vi "Command Channel.vi"(8 "error in":errorcluster, 11 "Node Ptr":T1 format="%.0x") -> (0 "error out":errorcluster)   [LabVIEW 2020, in "Ballard MIL-STD-1553 System Explorer.lvlib" / "Implementation.lvlib"]
uses:
  Implementation.lvlib
  <vilib>/NI VeriStand/Custom Device API/Custom Device Item Ref.ctl
  <vilib>/NI VeriStand/Custom Device API/Custom Device Channel Type.ctl
  <vilib>/NI VeriStand/Custom Device API/Custom Device API.lvlib
panel:
  out "Channel Settings":string[][](table)
  in  "Default Value":dbl
  in  "SHDocVw.IWebBrowser":refnum<k7>(container)
  in  "General Header":cluster{"Section Name":string}={"Section Name"="Ballard MIL-STD 1553 - Command Channel"}
  in  "Description":string
  out "Name":string
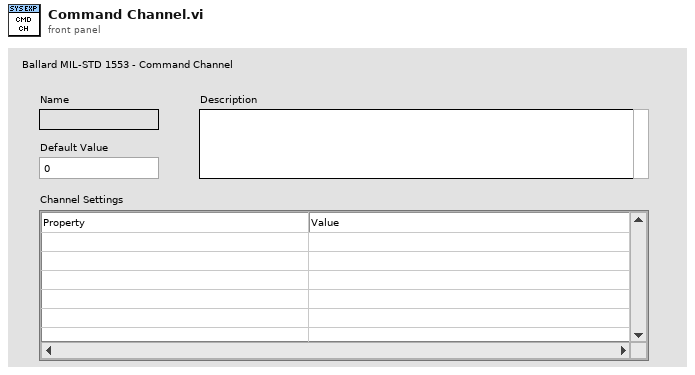
[diagram p1: front panel]
types:
  T1 = typedef "Custom Device API.lvlib/Custom Device Item Ref.ctl" = u64
  T2 = typedef "Custom Device API.lvlib/Custom Device Channel Type.ctl" = enum16{"Input", "Output"}
  T3 = typedef "Custom Device API.lvlib/Custom Device Channel.ctl" = cluster{"Type":T2, "Units":string, "Default Value":dbl, "Faultable":bool, "Scalable":bool}
  T4 = typedef "Custom Device API.lvlib/Custom Device Commands.ctl" = enum16{"Default", "Item renamed", "Shutdown", "Dynamic button pressed"}
  T5 = typedef "Custom Device API.lvlib/Custom Device Item Info.ctl" = cluster{"Name":string, "Is Channel":bool, "GUID":string, "Is Waveform":bool}
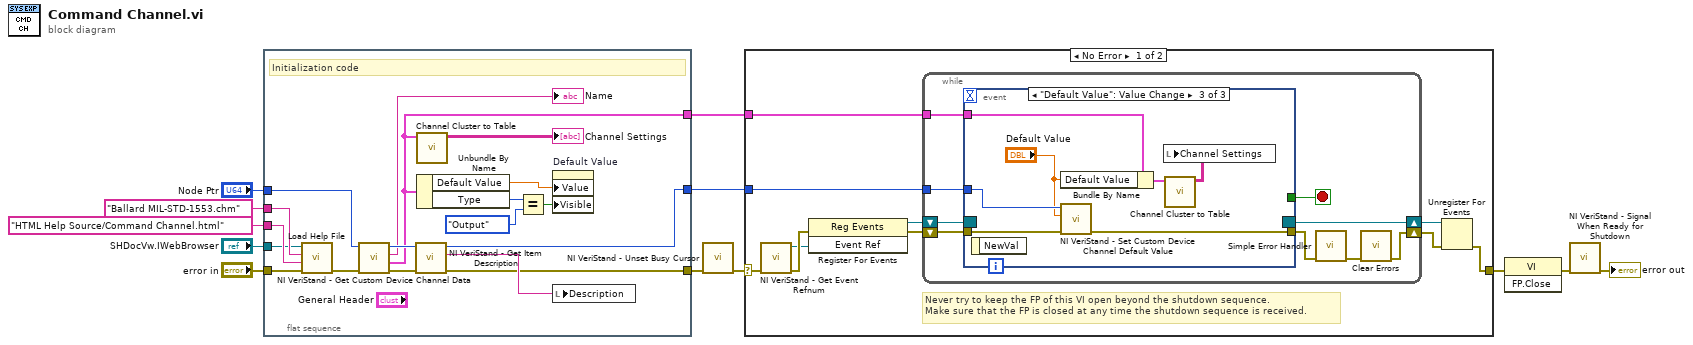
[diagram p0: block diagram]
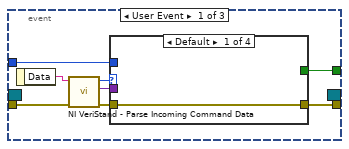
[diagram p2: hidden frame]
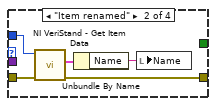
[diagram p3: hidden frame]
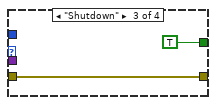
[diagram p4: hidden frame]
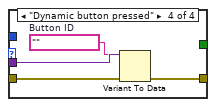
[diagram p5: hidden frame]
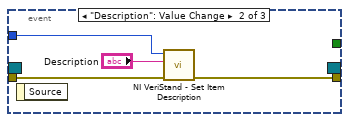
[diagram p6: hidden frame]
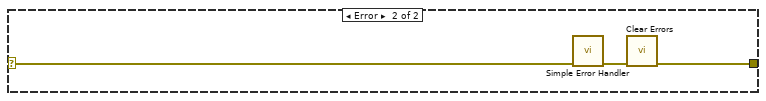
[diagram p7: hidden frame]
diagram:
  n1 = flat-sequence "Initialization code" {
    tunnel: "error in" -> [w29]
    tunnel: "Node Ptr" -> [w25]
    tunnel: [w24] -> w8
    tunnel: [w23] -> w5
    tunnel: "SHDocVw.IWebBrowser" -> [w26]
    tunnel: "HTML Help Source/Command Channel.html" ("CD_CHM_Section") -> [w28]
    tunnel: "Ballard MIL-STD-1553.chm" ("CD_CHM_FileName") -> [w27]
    tunnel: [w13] -> w1
    frame #0 {
      # "Initialization code"
      n2 = call "Load Help File.vi"("error in (no error)"=w29, "HTML File to Load"=w28, "Main CHM File"=w27, "Browser"=w26) -> ("error out"=w21:errorcluster)  [unwired: 7 in]
      n3 = call <vilib>:"NI VeriStand - Get Custom Device Channel Data.vi"("error in (no error)"=w21, "Channel Ref in"=w25) -> ("error out"=w22:errorcluster, "Channel"=w13:T3, "Channel Name"=→"Name":string, "Channel Ref out"=w17:T1)  [unwired: 4 in, 2 out]
      n4 = call <vilib>:"NI VeriStand - Get Item Description.vi"("error in (no error)"=w22, "Item Ref in"=w17) -> ("error out"=w24:errorcluster, "Description"=w30:string, "Item Ref out"=w23:T1)  [unwired: 7 out]
      n5 = call "Channel Cluster to Table.vi"("channel settings"=w13) -> ("channel settings table"=→"Channel Settings":string[][])  [unwired: 10 in]
      n6 = Unbundle By Name(w13) -> ("Default Value"=w14:dbl, "Type"=w20:T2)
      n7 = Equal?(x=w20, y=Custom_Device_Channel_Type."Output" ("x")) -> (x = y?=w18:bool)
      n8 = property on="Default Value" class="DigNum (strict)"("Value"=w14, "Visible"=w18) -> ()  [unwired: 2 in, 2 out]
      n9 = local write "Description"(w30) -> ()
    }
  }
  n10 = call <vilib>:"NI VeriStand - Unset Busy Cursor.vi"("error in (no error)"=w8) -> ("error out"=w7:errorcluster)  [unwired: 10 out]
  n11 = case shown="No Error" w7 {
    selector: w7 -> [w32 w83]
    tunnel: [w37 w81] -> w12
    tunnel: w5 -> [w33 _]
    tunnel: w1 -> [w31 _]
    frame No Error {
      # "Never try to keep the FP of this VI open beyond the shutdown sequence.\nMake sure that the FP is closed at any time the shutdown sequence is received."
      n12 = call <vilib>:"NI VeriStand - Get Event Refnum.vi"("error in (no error)"=w32) -> ("error out"=w40:errorcluster, "Event Ref"=w36:refnum<user-event>)  [unwired: 9 out]
      n13 = register-events(error in=w40, w36) -> (reference out=w34:refnum<event-registration>, error out=w35:errorcluster)  [unwired: 1 in]
      n14 = while {
        tunnel: w33 -> [w45]
        shift-right: [w42] -> w38
        shift-left: w35 -> [w48]
        shift-right: [w49] -> w39
        shift-left: w34 -> [w47]
        tunnel: w31 -> [w41]
        stop <- w46 stop-if-true
        n15 = event shown="[2] \"Default Value\": Value Change" {
          selector: w47 -> [_ _ _]
          dyn-events: [_ _ _] -> w49
          timeout: _ -> [_ _ _]
          tunnel: w48 -> [w57 w72 w80]
          tunnel: [w54 _ _] -> w46
          tunnel: [w53 w71 w79] -> w44
          tunnel: w45 -> [w52 w73 w78]
          tunnel: w41 -> [_ _ w76]
          event User Event {
            n16 = event-data() -> ("Data"=w50:string)  [unwired: 1 out]
            n17 = call <vilib>:"NI VeriStand - Parse Incoming Command Data.vi"("error in (no error)"=w57, "Incoming data"=w50) -> ("error out"=w56:errorcluster, "Outgoing data"=w51:variant, "Action"=w55:T4)  [unwired: 7 out]
            n18 = case shown="Default" w55 {
              tunnel: w56 -> [w58 w63 w64 w69]
              tunnel: [_ _ TRUE _] -> w54
              tunnel: [w58 w60 w64 w66] -> w53
              tunnel: w52 -> [_ w62 _ _]
              tunnel: w51 -> [_ _ _ w68]
              frame Default {
              }
              frame "Item renamed" {
                n19 = call <vilib>:"NI VeriStand - Get Item Data.vi"("error in (no error)"=w63, "Item Ref in"=w62) -> ("error out"=w60:errorcluster, "Item Info"=w61:T5)  [unwired: 8 out]
                n20 = Unbundle By Name(w61) -> ("Name"=w59:string)
                n21 = local write "Name"(w59) -> ()
              }
              frame "Shutdown" {
              }
              frame "Dynamic button pressed" {
                w67 = ""  # Button ID
                n22 = Variant To Data(error in=w69, type=w67, Variant=w68) -> (error out=w66:errorcluster)  [unwired: 1 out]
              }
            }
          }
          event "Description": Value Change {
            n23 = event-data() -> ()  [unwired: 2 out]
            n24 = call <vilib>:"NI VeriStand - Set Item Description.vi"("error in (no error)"=w72, "Description"="Description", "Item Ref in"=w73) -> ("error out"=w71:errorcluster)  [unwired: 8 out]
          }
          event "Default Value": Value Change {
            n25 = event-data() -> ()  [unwired: 2 out]
            n26 = Bundle By Name(cluster=w76, "Default Value"="Default Value") -> (w74:T3)
            n27 = call <vilib>:"NI VeriStand - Set Custom Device Channel Default Value.vi"("error in (no error)"=w80, "Default Value"="Default Value", "Channel Ref in"=w78) -> ("error out"=w79:errorcluster)  [unwired: 7 in, 1 out]
            n28 = call "Channel Cluster to Table.vi"("channel settings"=w74) -> ("channel settings table"=w77:string[][])  [unwired: 10 in]
            n29 = local write "Channel Settings"(w77) -> ()
          }
        }
        n30 = call <vilib>:"Simple Error Handler.vi"("error in (no error)"=w44) -> ("error out"=w43:errorcluster)  [unwired: 1 in, 7 out]
        n31 = call <vilib>:"Clear Errors.vi"("error in (no error)"=w43) -> ("error out"=w42:errorcluster)  [unwired: 1 in, 5 out]
      }
      n32 = Unregister For Events(event registration refnum=w39, error in=w38) -> (error out=w37:errorcluster)
    }
    frame Error {
      n33 = call <vilib>:"Simple Error Handler.vi"("error in (no error)"=w83) -> ("error out"=w82:errorcluster)  [unwired: 1 in, 7 out]
      n34 = call <vilib>:"Clear Errors.vi"("error in (no error)"=w82) -> ("error out"=w81:errorcluster)  [unwired: 1 in, 5 out]
    }
  }
  n35 = invoke class="VI" method="FP.Close"(error in=w12) -> (error out=w11:errorcluster)  [unwired: 2 in, 2 out]
  n36 = call <vilib>:"NI VeriStand - Signal When Ready for Shutdown.vi"("error in (no error)"=w11) -> ("error out"=→"error out":errorcluster)  [unwired: 10 out]
